vi "Main.vi"() -> ()   [LabVIEW 2016]
uses:
  Experiment States.ctl
  <vilib>/DAQmx/read.llb/DAQmx Read (Analog 2D DBL NChan NSamp).vi
  <vilib>/DAQmx/read.llb/DAQmx Read (Analog 1D DBL 1Chan NSamp).vi
  <vilib>/DAQmx/miscellaneous.llb/DAQmx Fill In Error Info.vi
panel:
  in  "Thermocouple 5 Type":i32(ring)=10073 items=["J"=10072, "K"=10073, "N"=10077, "R"=10082, "S"=10085, "T"=10086, "B"=10047, "E"=10055]
  in  "Thermocouple 4 Type":i32(ring)=10073 items=["J"=10072, "K"=10073, "N"=10077, "R"=10082, "S"=10085, "T"=10086, "B"=10047, "E"=10055]
  in  "Thermocouple 3 Type":i32(ring)=10073 items=["J"=10072, "K"=10073, "N"=10077, "R"=10082, "S"=10085, "T"=10086, "B"=10047, "E"=10055]
  in  "Thermocouple 2 Type":i32(ring)=10073 items=["J"=10072, "K"=10073, "N"=10077, "R"=10082, "S"=10085, "T"=10086, "B"=10047, "E"=10055]
  in  "Thermocouple 1 Type":i32(ring)=10073 items=["J"=10072, "K"=10073, "N"=10077, "R"=10082, "S"=10085, "T"=10086, "B"=10047, "E"=10055]
  out "Thermocouple Graph":cluster{"X":dbl, "Y":dbl}[](graph)
  out "Conductivity Meter Graph":cluster{"X":dbl, "Y":dbl}[](graph)
  out "Thermocouple 5":dbl(slide) scale=0.0..50.0
  out "Thermocouple 4":dbl(slide) scale=0.0..50.0
  out "Thermocouple 3":dbl(slide) scale=0.0..50.0
  out "Thermocouple 2":dbl(slide) scale=0.0..50.0
  out "Thermocouple 1":dbl(slide) scale=0.0..50.0
  in  "Thermocouple 5 Channel":tag
  in  "Thermocouple 4 Channel":tag
  in  "Thermocouple 3 Channel":tag
  in  "Thermocouple 2 Channel":tag
  in  "Thermocouple 1 Channel":tag
  in  "Conductivity Meter Channel":tag
  in  "Skip Export":bool
  in  "End Experiment?":bool
  in  "Export?":bool
  in  "Start":bool
  # "The above values need to be set before the experiment is started"
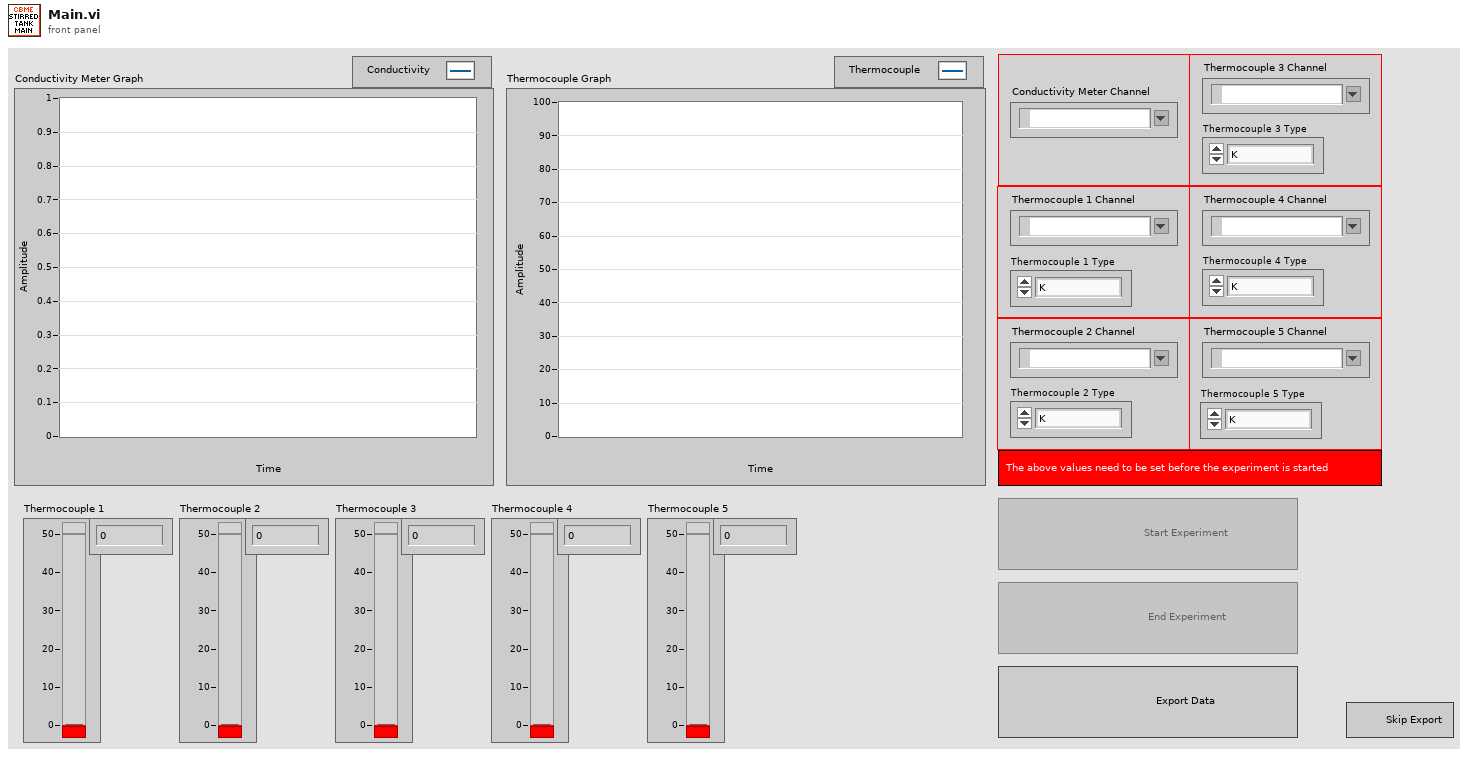
[diagram p1: front panel]
types:
  T1 = typedef "Experiment States.ctl" = enum16{"Setup", "Data Collection", "Export", "Finish"}
  T2 = enum8{"Enabled", "Disabled", "Disabled and Grayed Out"}
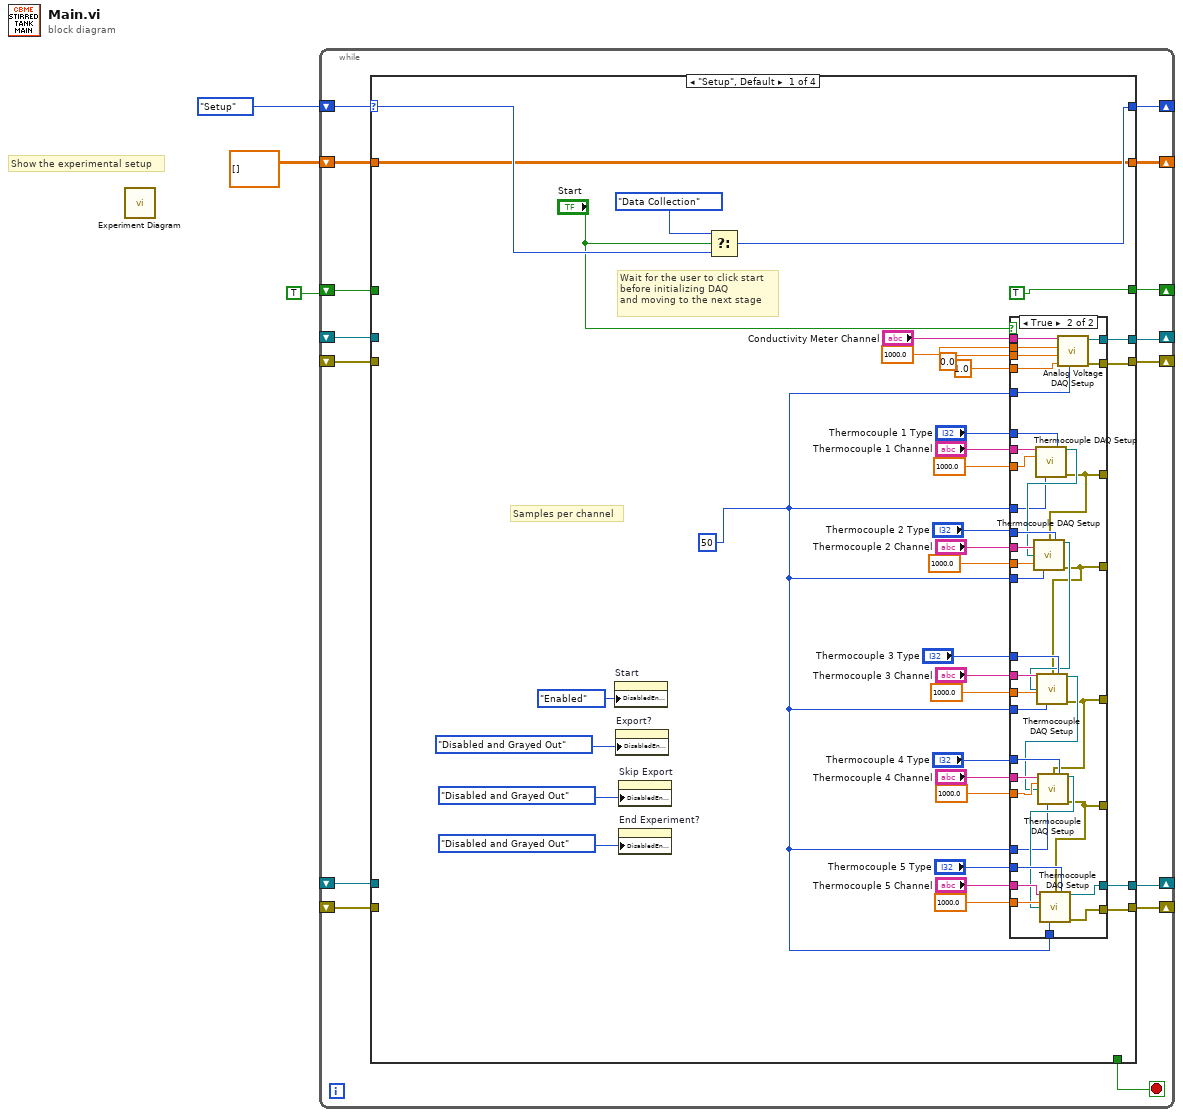
[diagram p0: block diagram]
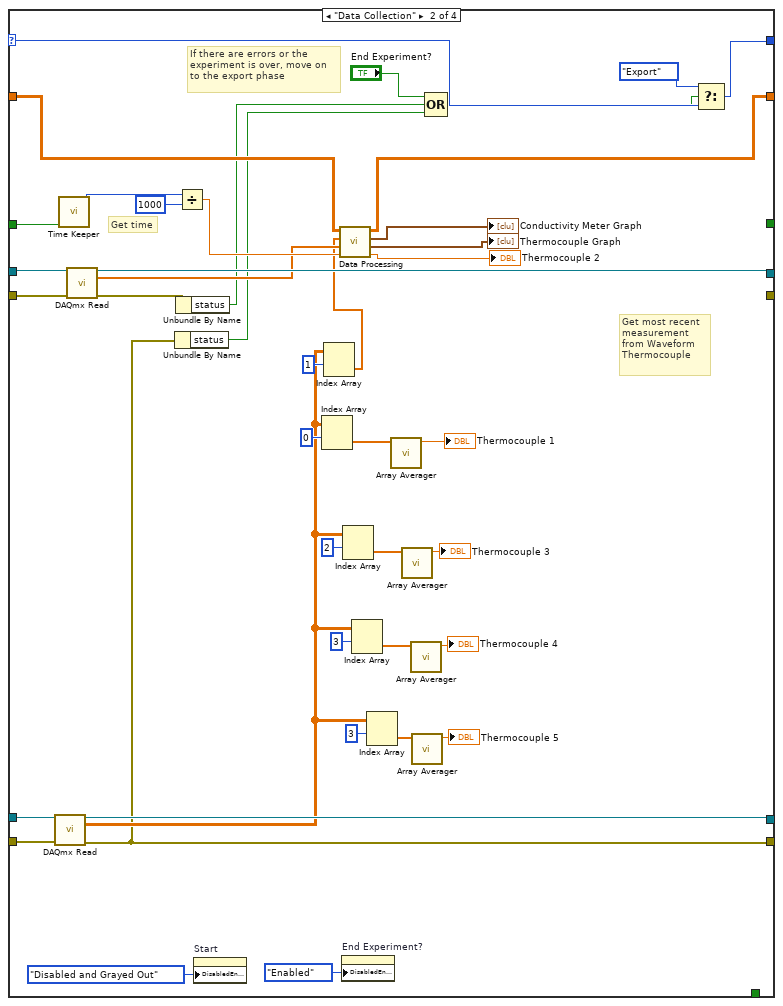
[diagram p3: hidden frame]
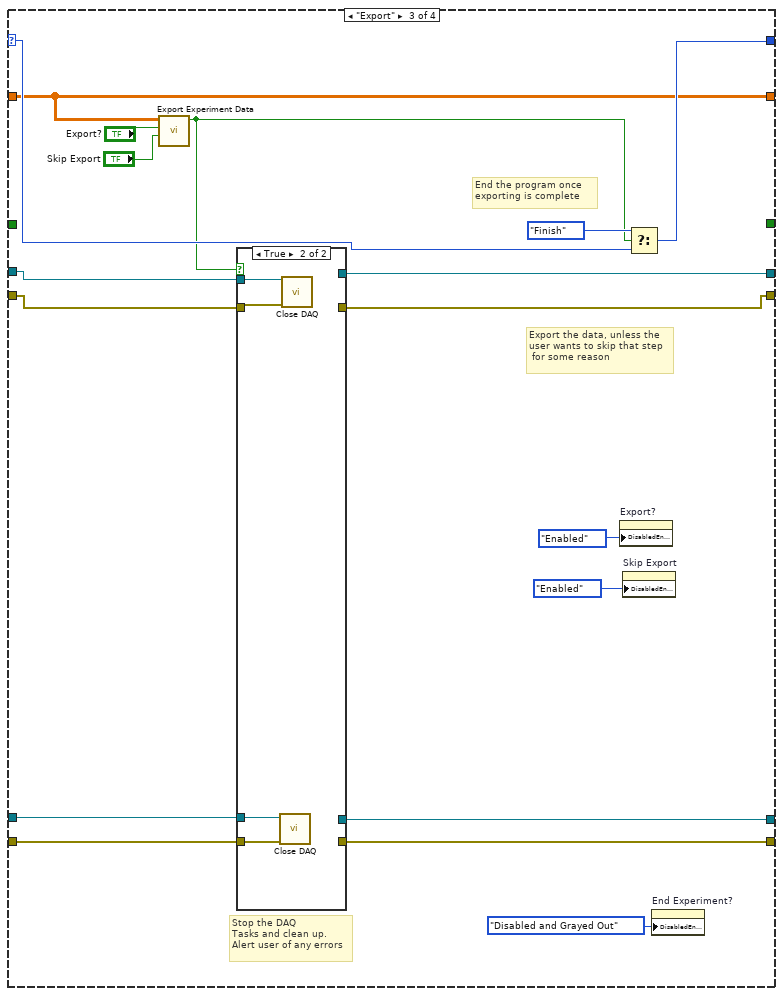
[diagram p4: hidden frame]
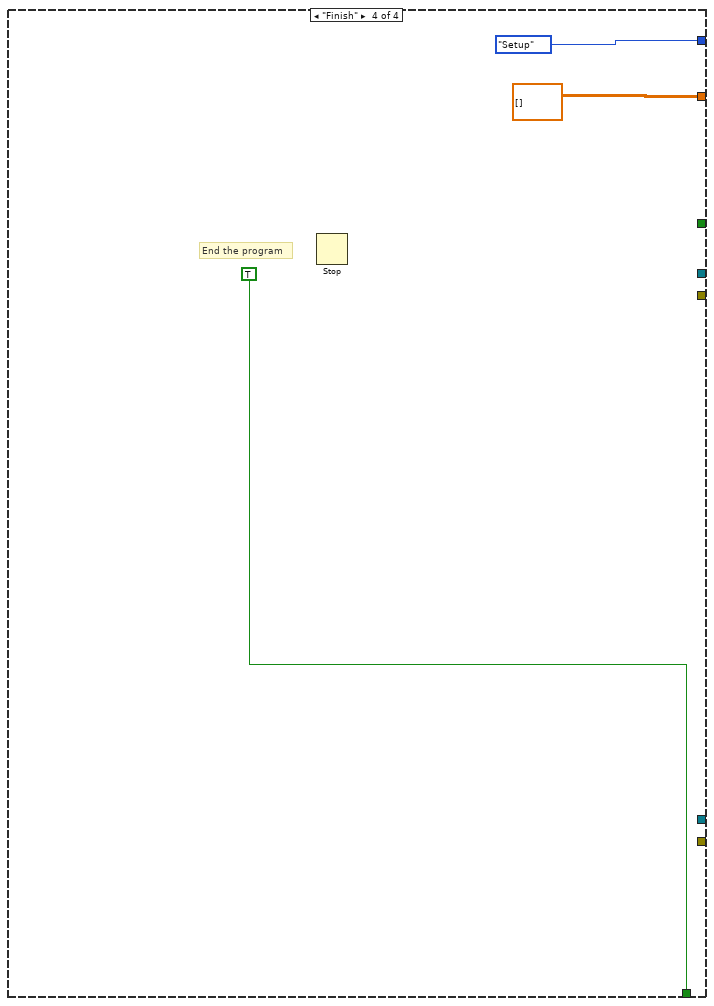
[diagram p6: hidden frame]
diagram:
  # "Show the experimental setup"
  n1 = call "Experiment Diagram.vi"() -> ()  [unwired: 12 in]
  n2 = while {
    shift-right: [w17] -> _
    shift-left: Experiment_States."Setup" -> [w18]
    shift-right: [w10] -> _
    shift-left: dbl[][] [] -> [w11]
    shift-right: [w8] -> _
    shift-left: TRUE -> [w9]
    shift-right: [w7] -> _
    shift-left: _ -> [w14]
    shift-right: [w6] -> _
    shift-left: _ -> [w12]
    shift-right: [w4] -> _
    shift-left: _ -> [w13]
    shift-right: [w5] -> _
    shift-left: _ -> [w15]
    stop <- w16 stop-if-true
    n3 = case shown="\"Setup\", Default" w18 {
      selector: w18 -> [w52 w127 w149 _]
      tunnel: [w50 w125 w145 Experiment_States."Setup"] -> w17
      tunnel: [_ _ _ TRUE] -> w16
      tunnel: w15 -> [_ w131 w140 _]
      tunnel: w14 -> [_ w130 w139 _]
      tunnel: w13 -> [_ w129 w138 _]
      tunnel: w12 -> [_ w128 w137 _]
      tunnel: w11 -> [w49 w115 w144 _]
      tunnel: [w49 w114 w144 dbl[][] []] -> w10
      tunnel: w9 -> [_ w122 _ _]
      tunnel: [TRUE _ _ _] -> w8
      tunnel: [w28 _ w135 _] -> w7
      tunnel: [w26 w92 w133 _] -> w6
      tunnel: [w27 w117 w136 _] -> w5
      tunnel: [w25 w116 w134 _] -> w4
      frame "Setup", Default {
        w19 = 50
        # "Samples per channel"
        # "Wait for the user to click start \nbefore initializing DAQ\nand moving to the next stage"
        n4 = property on="Start" class="Bool"("DisabledEnum"=T2."Enabled" ("Disabled")) -> ()  [unwired: 2 in, 2 out]
        n5 = property on="Export?" class="Bool"("DisabledEnum"=T2."Disabled and Grayed Out" ("Disabled")) -> ()  [unwired: 2 in, 2 out]
        n6 = property on="Skip Export" class="Bool"("DisabledEnum"=T2."Disabled and Grayed Out" ("Disabled")) -> ()  [unwired: 2 in, 2 out]
        n7 = property on="End Experiment?" class="Bool"("DisabledEnum"=T2."Disabled and Grayed Out" ("Disabled")) -> ()  [unwired: 2 in, 2 out]
        n8 = Select(t=Experiment_States."Data Collection", s="Start", f=w52) -> (s? t:f=w50:T1)
        n9 = case shown="True" "Start" {
          tunnel: [_ w89] -> w27
          tunnel: [_ w88] -> w28
          tunnel: [_ w62] -> _
          tunnel: [_ w61] -> _
          tunnel: [_ w60] -> _
          tunnel: [_ w59] -> _
          tunnel: [_ w87] -> w25
          tunnel: [_ w86] -> w26
          tunnel: "Conductivity Meter Channel" -> [_ w85]
          tunnel: 1000.0 ("Sample Rate") -> [_ w84]
          tunnel: 0.0 ("minimum value") -> [_ w83]
          tunnel: 1.0 ("maximum value") -> [_ w82]
          tunnel: "Thermocouple 1 Channel" -> [_ w81]
          tunnel: 1000.0 ("Sample Rate") -> [_ w80]
          tunnel: "Thermocouple 1 Type" -> [_ w79]
          tunnel: "Thermocouple 2 Type" -> [_ w78]
          tunnel: "Thermocouple 2 Channel" -> [_ w77]
          tunnel: 1000.0 ("Sample Rate") -> [_ w76]
          tunnel: "Thermocouple 3 Type" -> [_ w75]
          tunnel: "Thermocouple 3 Channel" -> [_ w74]
          tunnel: 1000.0 ("Sample Rate") -> [_ w73]
          tunnel: "Thermocouple 4 Type" -> [_ w72]
          tunnel: "Thermocouple 4 Channel" -> [_ w71]
          tunnel: 1000.0 ("Sample Rate") -> [_ w70]
          tunnel: "Thermocouple 5 Type" -> [_ w69]
          tunnel: "Thermocouple 5 Channel" -> [_ w68]
          tunnel: 1000.0 ("Sample Rate") -> [_ w67]
          tunnel: w19 -> [_ w58]
          tunnel: w19 -> [_ w57]
          tunnel: w19 -> [_ w56]
          tunnel: w19 -> [_ w55]
          tunnel: w19 -> [_ w54]
          tunnel: w19 -> [_ w53]
          frame False {
          }
          frame True {
            n10 = call "Thermocouple DAQ Setup.vi"("physical channels"=w81, "Thermocouple Type"=w79, "Sample Rate"=w80, "samples per channel"=w58) -> ("task out"=w66:refnum<k21>, "error out"=w62:errorcluster)  [unwired: 10 in]
            n11 = call "Thermocouple DAQ Setup.vi"("physical channels"=w77, "error in"=w62, "Thermocouple Type"=w78, "Sample Rate"=w76, "task in"=w66, "samples per channel"=w57) -> ("task out"=w65:refnum<k21>, "error out"=w61:errorcluster)  [unwired: 8 in]
            n12 = call "Thermocouple DAQ Setup.vi"("physical channels"=w74, "error in"=w61, "Thermocouple Type"=w75, "Sample Rate"=w73, "task in"=w65, "samples per channel"=w56) -> ("task out"=w64:refnum<k21>, "error out"=w60:errorcluster)  [unwired: 8 in]
            n13 = call "Thermocouple DAQ Setup.vi"("physical channels"=w71, "error in"=w60, "Thermocouple Type"=w72, "Sample Rate"=w70, "task in"=w64, "samples per channel"=w55) -> ("task out"=w63:refnum<k21>, "error out"=w59:errorcluster)  [unwired: 8 in]
            n14 = call "Thermocouple DAQ Setup.vi"("physical channels"=w68, "error in"=w59, "Thermocouple Type"=w69, "Sample Rate"=w67, "task in"=w63, "samples per channel"=w54) -> ("task out"=w87:refnum<k21>, "error out"=w86:errorcluster)  [unwired: 8 in]
            n15 = call "Analog Voltage DAQ Setup.vi"("samples per channel"=w53, "maximum value"=w82, "minimum value"=w83, "Sample Rate"=w84, "physical channels"=w85) -> ("error out"=w88:errorcluster, "task out"=w89:refnum<k21>)  [unwired: 5 in]
          }
        }
      }
      frame "Data Collection" {
        # "If there are errors or the \nexperiment is over, move on\nto the export phase"
        # "Get time"
        # "Get most recent \nmeasurement \nfrom Waveform\nThermocouple"
        n16 = call-poly <vilib>:"DAQmx Read.vi"("task/channels in"=w129, "error in"=w128) -> ("task out"=w116:refnum<k21>, "data"=w95:dbl[][], "error out"=w92:errorcluster)  [unwired: 11 in]
        n17 = call "Time Keeper.vi"("Reset?"=w122) -> ("Time Elapsed (ms)"=w121:u32)  [unwired: 10 in]
        n18 = call-poly <vilib>:"DAQmx Read.vi"("task/channels in"=w131, "error in"=w130) -> ("task out"=w117:refnum<k21>, "data"=w112:dbl[], "error out"=w93:errorcluster)  [unwired: 11 in]
        n19 = Unbundle By Name(w92) -> ("status"=w90:bool)
        n20 = Unbundle By Name(w93) -> ("status"=w91:bool)
        n21 = Divide(x=w121, y=u32 1000) -> (x/y=w113:dbl)
        n22 = property on="Start" class="Bool"("DisabledEnum"=T2."Disabled and Grayed Out" ("Disabled")) -> ()  [unwired: 2 in, 2 out]
        n23 = Index Array(array=w95, index (row)=0) -> (element=w107:dbl[])  [unwired: 1 in]
        n24 = Index Array(array=w95, index (row)=1) -> (element=w104:dbl[])  [unwired: 1 in]
        n25 = call "Data Processing.vi"("Time"=w113, "Conductivity Array"=w112, "Thermocouple 2 Array"=w104, "Data in"=w115) -> ("Most Recent T2"=→"Thermocouple 2":dbl, "Thermocouple Graph"=→"Thermocouple Graph":cluster{"X":dbl, "Y":dbl}[], "Conductivity Meter Graph"=→"Conductivity Meter Graph":cluster{"X":dbl, "Y":dbl}[], "Data out"=w114:dbl[][])  [unwired: 4 in]
        n26 = property on="End Experiment?" class="Bool"("DisabledEnum"=T2."Enabled" ("Disabled")) -> ()  [unwired: 2 in, 2 out]
        n27 = Index Array(array=w95, index (row)=2) -> (element=w102:dbl[])  [unwired: 1 in]
        n28 = Index Array(array=w95, index (row)=3) -> (element=w100:dbl[])  [unwired: 1 in]
        n29 = Index Array(array=w95, index (row)=3) -> (element=w96:dbl[])  [unwired: 1 in]
        n30 = call "Array Averager.vi"("Array"=w107) -> ("Averaged Array"=→"Thermocouple 1":dbl)  [unwired: 10 in]
        n31 = call "Array Averager.vi"("Array"=w102) -> ("Averaged Array"=→"Thermocouple 3":dbl)  [unwired: 10 in]
        n32 = call "Array Averager.vi"("Array"=w100) -> ("Averaged Array"=→"Thermocouple 4":dbl)  [unwired: 10 in]
        n33 = call "Array Averager.vi"("Array"=w96) -> ("Averaged Array"=→"Thermocouple 5":dbl)  [unwired: 10 in]
        n34 = Compound Arithmetic op=OR("End Experiment?", w91, w90) -> (w118:bool)
        n35 = Select(t=Experiment_States."Export", s=w118, f=w127) -> (s? t:f=w125:T1)
      }
      frame "Export" {
        # "End the program once \nexporting is complete"
        # "Export the data, unless the \nuser wants to skip that step\n for some reason"
        # "Stop the DAQ \nTasks and clean up.\nAlert user of any errors"
        n36 = call "Export Experiment Data.vi"("Skip Export"="Skip Export", "Export?"="Export?", "Data"=w144) -> ("Export Complete?"=w141:bool)  [unwired: 8 in]
        n37 = case shown="True" w141 {
          tunnel: w140 -> [w153 w157]
          tunnel: w139 -> [w152 w156]
          tunnel: w138 -> [w151 w155]
          tunnel: w137 -> [w150 w154]
          tunnel: [w153 _] -> w136
          tunnel: [w152 _] -> w135
          tunnel: [w151 _] -> w134
          tunnel: [w150 _] -> w133
          frame False {
          }
          frame True {
            n38 = call "Close DAQ.vi"("error in (no error)"=w154, "Refnum in"=w155) -> ()  [unwired: 10 in]
            n39 = call "Close DAQ.vi"("error in (no error)"=w156, "Refnum in"=w157) -> ()  [unwired: 10 in]
          }
        }
        n40 = property on="Export?" class="Bool"("DisabledEnum"=T2."Enabled" ("Disabled")) -> ()  [unwired: 2 in, 2 out]
        n41 = property on="Skip Export" class="Bool"("DisabledEnum"=T2."Enabled" ("Disabled")) -> ()  [unwired: 2 in, 2 out]
        n42 = Select(t=Experiment_States."Finish", s=w141, f=w149) -> (s? t:f=w145:T1)
        n43 = property on="End Experiment?" class="Bool"("DisabledEnum"=T2."Disabled and Grayed Out" ("Disabled")) -> ()  [unwired: 2 in, 2 out]
      }
      frame "Finish" {
        # "End the program"
        n44 = Stop() -> ()  [unwired: 1 in]
      }
    }
  }
